vi "SVD Generalise.vi"() -> ()   [LabVIEW 2017]
uses:
  <vilib>/Analysis/Matrix/Datatypes/RealMatrix.ctl
  <vilib>/Analysis/7linalg.llb/SVD Option.ctl
  <vilib>/Analysis/7linalg.llb/Real Generalized SVD Decomposition.vi
  <vilib>/Analysis/NI_AALPro.lvlib
  <vilib>/Analysis/Matrix/NI_Matrix.lvlib
panel:
  out "Saving Data 2":bool caption="Saving Data"
  out "Saving Data":bool
  in  "?":bool
  out "Matrix S":T1
  out "Matrix C":T1
  out "Matrix R":T1
  out "Matrix V":T1
  out "Matrix U":T1
  out "Singular Values":dbl[](array[numeric])
  in  "SVD option":T2 items=["Thin", "Full"]
  in  "singular values only?":bool
  in  "B":T1
  in  "A":T1
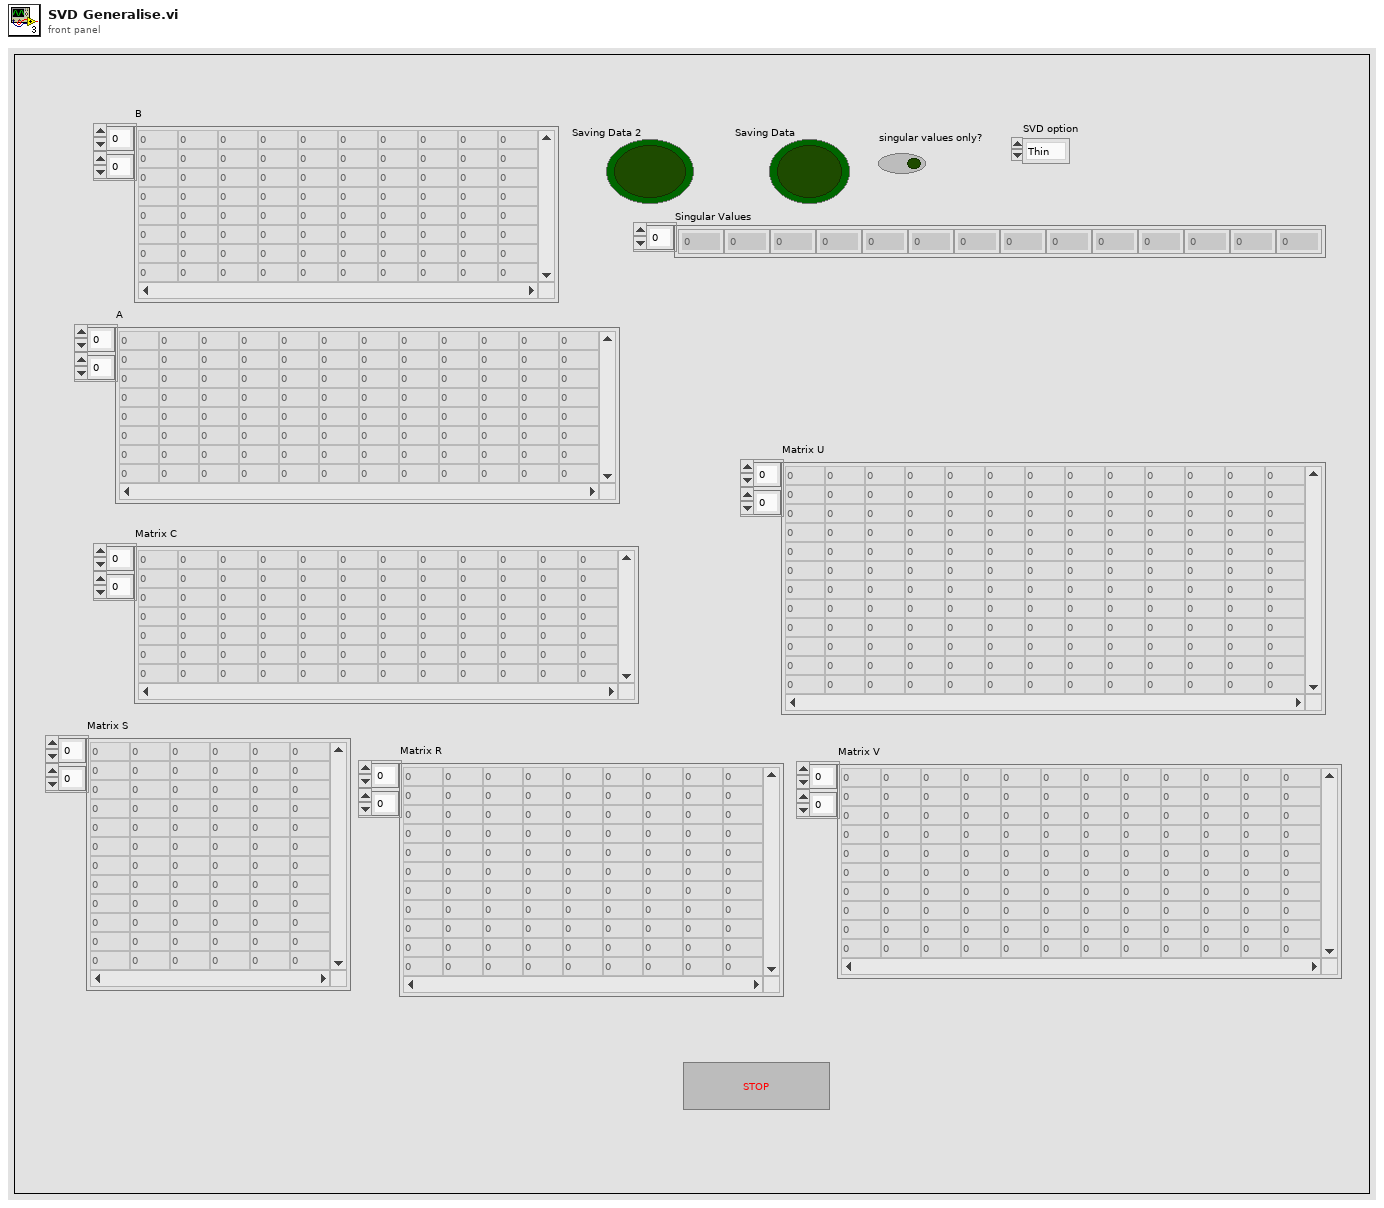
[diagram p1: front panel]
types:
  T1 = typedef "NI_Matrix.lvlib/RealMatrix.ctl" = dbl[][]
  T2 = typedef "NI_AALPro.lvlib/SVD Option.ctl" = u16
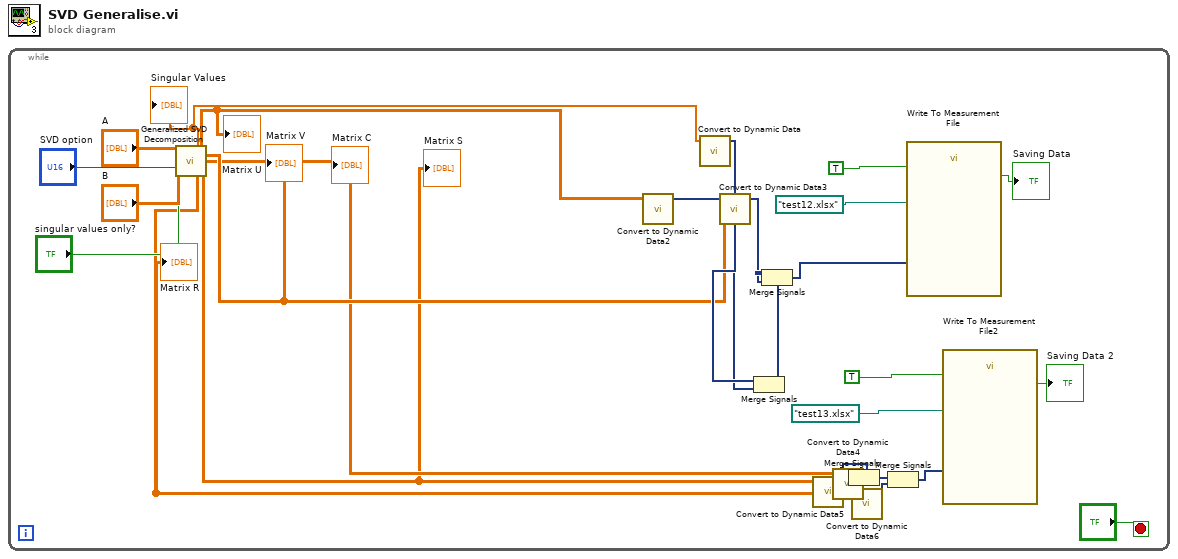
[diagram p0: block diagram]
diagram:
  n1 = while {
    stop <- "?" stop-if-true
    n2 = call-poly <vilib>:"Generalized SVD Decomposition.vi"("A"="A", "B"="B", "singular values only?"="singular values only?", "SVD option"="SVD option") -> ("Singular Values"=w22:dbl[], "Matrix U"=w19:T1, "Matrix V"=w16:T1, "Matrix C"=w9:T1, "Matrix S"=w6:T1, "Matrix R"=w3:T1)  [unwired: 5 in, 1 out]
    "Singular Values" <- w22
    "Matrix U" <- w19
    "Matrix V" <- w16
    "Matrix R" <- w3
    "Matrix C" <- w9
    "Matrix S" <- w6
    n3 = call "Convert to Dynamic Data2"("2D Array"=w19) -> ("Dynamic Data Type"=w18:dynamicdata)  [unwired: 3 in]
    n4 = call "Convert to Dynamic Data"("Array"=w22) -> ("Dynamic Data Type"=w21:dynamicdata)  [unwired: 3 in]
    n5 = call "Convert to Dynamic Data3"("2D Array"=w16) -> ("Dynamic Data Type"=w15:dynamicdata)  [unwired: 3 in]
    n6 = Merge Signals(w21, w18) -> (w20:dynamicdata)
    n7 = Merge Signals(w20, w15) -> (w17:dynamicdata)
    n8 = call "Convert to Dynamic Data5"("2D Array"=w6) -> ("Dynamic Data Type"=w5:dynamicdata)  [unwired: 3 in]
    n9 = call "Convert to Dynamic Data4"("2D Array"=w9) -> ("Dynamic Data Type"=w8:dynamicdata)  [unwired: 3 in]
    n10 = Merge Signals(w8, w5) -> (w7:dynamicdata)
    n11 = call "Convert to Dynamic Data6"("2D Array"=w3) -> ("Dynamic Data Type"=w2:dynamicdata)  [unwired: 3 in]
    n12 = Merge Signals(w7, w2) -> (w4:dynamicdata)
    n13 = call "Write To Measurement File"("Signals"=w17, "Enable"=TRUE, "Filename"=path "test12.xlsx") -> ("Saving Data"=→"Saving Data":bool)  [unwired: 14 in, 2 out]
    n14 = call "Write To Measurement File2"("Signals"=w4, "Enable"=TRUE, "Filename"=path "test13.xlsx") -> ("Saving Data"=→"Saving Data 2":bool)  [unwired: 14 in, 2 out]
  }
